vi "ziListDevices.vi"(4 "Error In":errorcluster, 7 "Handle In":T1 {"Handle" format="0x%08x"; "Conn" format="0x%08x"}) -> (0 "Error Out":errorcluster, 2 "Devices":cluster{"Nodes":string, i32}[](array[cluster]), 3 "Handle Out":T1 {"Handle" format="0x%08x"; "Conn" format="0x%08x"})   [LabVIEW 2009, in "Zurich Instruments LabOne.lvlib"]
doc: "Returns a list of ZI Instruments that are available in the connected Data Server."
uses:
  <instrlib>/Zurich Instruments LabOne/Zurich Instruments LabOne.lvlib
  <instrlib>/Zurich Instruments LabOne/Public/ziTypeHandle.ctl
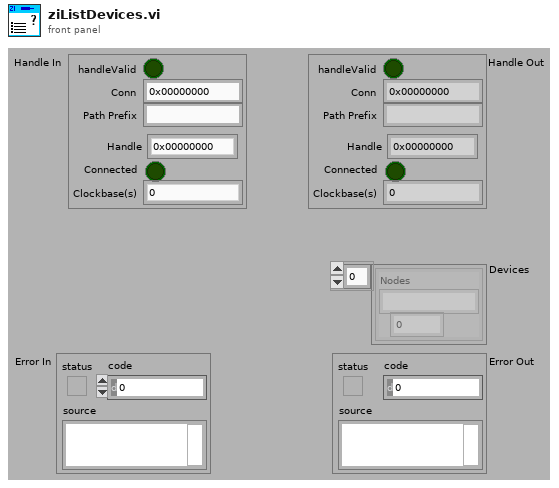
[diagram p1: front panel]
types:
  T1 = typedef "Zurich Instruments LabOne.lvlib/ziTypeHandle.ctl" = cluster{"handleValid":bool, "Conn":u64, "Path Prefix":string, "Handle":u64, "Connected":bool, "Clockbase(s)":dbl}
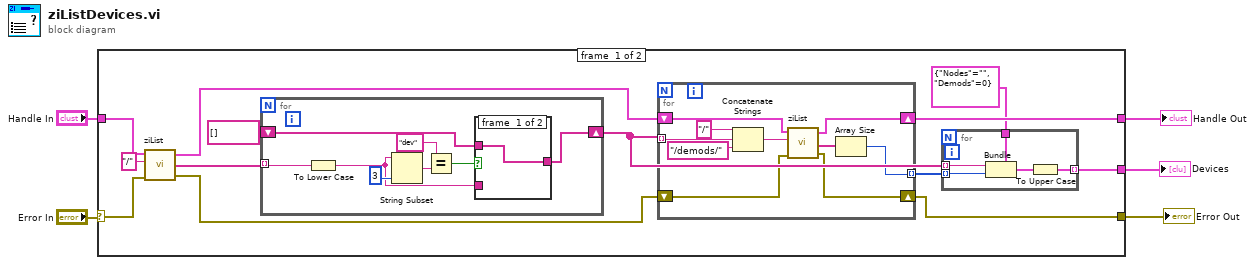
[diagram p0: block diagram]
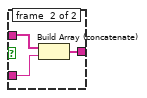
[diagram p2: hidden frame]
diagram:
  n1 = case shown="No Error" "Error In" {
    selector: "Error In" -> [w6 w47]
    tunnel: "Handle In" -> [w17 w46]
    tunnel: [w15 w46] -> w4
    tunnel: [w14 w47] -> w3
    tunnel: [w11 _] -> w2
    frame #0 {
      n2 = call <instrlib>:"ziList.vi"("Error In"=w6, "Path (\"\")"="/" ("Path (\"\")"), "Handle In"=w17) -> ("Error Out"=w10:errorcluster, "Nodes"=w16:string[], "Handle Out"=w9:T1)  [unwired: 1 out]
      n3 = for {
        tunnel: w16 -> [w35] mode=indexing
        shift-right: [w37] -> w13
        shift-left: string[] [] -> [w38]
        n4 = To Lower Case(string=w35) -> (all lower case string=w34:string)
        n5 = String Subset(string=w34, length (rest)=3 ("length (rest)")) -> (substring=w41:string)  [unwired: 1 out]
        n6 = Equal?(x="dev", y=w41) -> (x = y?=w39:bool)
        n7 = case shown="True" w39 {
          tunnel: w34 -> [_ w44]
          tunnel: w38 -> [w42 w45]
          tunnel: [w42 w43] -> w37
          frame #0 {
          }
          frame #1 {
            n8 = Build Array (concatenate)(w45, w44) -> (w43:string[])
          }
        }
      }
      n9 = for {
        tunnel: w13 -> [w32] mode=indexing
        shift-right: [w26] -> w15
        shift-left: w9 -> [w29]
        shift-right: [w28] -> w14
        shift-left: w10 -> [w27]
        tunnel: [w24] -> w12 mode=indexing
        n10 = Concatenate Strings("/" ("x"), w32, "/demods/" ("x")) -> (w30:string)
        n11 = call <instrlib>:"ziList.vi"("Error In"=w27, "Path (\"\")"=w30, "Handle In"=w29) -> ("Error Out"=w28:errorcluster, "Nodes"=w25:string[], "Handle Out"=w26:T1)  [unwired: 1 out]
        n12 = Array Size(array=w25) -> (size(s)=w24:i32)
      }
      n13 = for {
        tunnel: w13 -> [w23] mode=indexing
        tunnel: w12 -> [w22] mode=indexing
        tunnel: [w19] -> w11 mode=indexing
        tunnel: cluster{"Nodes":string, "Demods":i32} {"Nodes"="", "Demods"=0} ("cluster") -> [w21]
        n14 = Bundle(cluster=w21, "Nodes"=w23, "Demods"=w22) -> (w20:cluster{"Nodes":string, "Demods":i32})
        n15 = To Upper Case(1:w20) -> (0:w19:cluster{"Nodes":string, "Demods":i32})
      }
    }
    frame #1 {
    }
  }
  "Handle Out" <- w4
  "Error Out" <- w3
  "Devices" <- w2
